vi "Read Name.vi"(8 "Error In":errorcluster, 11 "Known Host In":refnum<class "Known Host.lvclass">) -> (0 "Error Out":errorcluster, 2 "Name":string, 3 "Known Host Out":refnum<class "Known Host.lvclass">)   [LabVIEW 2018, in "Toolkit.lvlib" / "Known Host.lvclass"]
uses:
  Known Host.lvclass
  Known Host.lvclass/Known Host.ctl
  SSH/SSH.lvclass/SSH.ctl
  Toolkit.lvlib
  SSH/SSH.lvclass
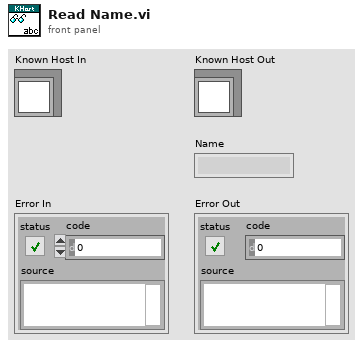
[diagram p1: front panel]
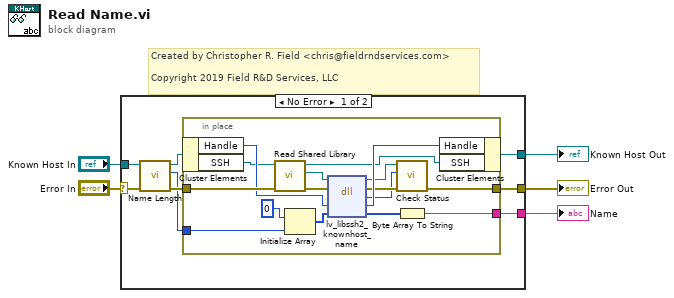
[diagram p0: block diagram]
diagram:
  # "Created by Christopher R. Field <chris@fieldrndservices.com>\n\nCopyright 2019 Field R&D Services, LLC"
  n1 = case shown="No Error" "Error In" {
    selector: "Error In" -> [w11 w31]
    tunnel: [w13 w31] -> w4
    tunnel: "Known Host In" -> [w9 w30]
    tunnel: [w12 w30] -> w2
    tunnel: [w6 _] -> w1
    frame No Error {
      n2 = call "Name Length.vi"("Error In"=w11, "Known Host In"=w9) -> ("Error Out"=w10:errorcluster, "Length"=w7:u64, "Known Host Out"=w8:refnum<class "Known Host.lvclass">)  [unwired: 7 in]
      n3 = in-place {
        in-place-border: w10 -> [w29]
        in-place-border: [w25] -> w13
        in-place-border: w7 -> [w21]
        in-place-border: [w18] -> w6
        n4 = in-place-cluster #1(w8) -> ("Handle"=w28:u64, "SSH"=w16:refnum<class "SSH.lvclass">)
        n5 = call "Read Shared Library.vi"("Error In"=w29, "SSH In"=w16) -> ("Error Out"=w17:errorcluster, "lv-libssh2 Shared Library"=w14:path, "SSH Out"=w15:refnum<class "SSH.lvclass">)  [unwired: 7 in]
        n6 = Initialize Array(u8 0, w21) -> (w20:u8[])
        n7 = dll-call lib="lv-libssh2.*" fn="lv_libssh2_knownhost_name"(path in=w14, error in=w17, "handle"=w28, "buffer"=w20) -> (path out=w24:path, error out=w26:errorcluster, "status"=w23:i32, "handle"=w27:u64, "buffer"=w19:u8[])  [unwired: 1 in]
        n8 = call "Check Status.vi"("Error In"=w26, "Status"=w23, "lv-libssh2 Shared Library In"=w24) -> ("Error Out"=w25:errorcluster)  [unwired: 7 in, 1 out]
        n9 = Byte Array To String(unsigned byte array=w19) -> (string=w18:string)
        n10 = in-place-cluster #1("Handle"=w27, "SSH"=w15) -> (w12:refnum<class "Known Host.lvclass">)
      }
    }
    frame Error {
    }
  }
  "Error Out" <- w4
  "Known Host Out" <- w2
  "Name" <- w1
